vi "SET_8BITS_Command.vi"(9 "Valor en 8 bits":u8, 10 "Marca":T1) -> (1 "length":i32, 2 "Expected Response":string, 3 "Command":string, 4 "Bytes Expected":u32=2)   [LabVIEW 2019, in "Serial Device.lvclass"]
uses:
  Serial Device.lvclass
  Marca.ctl
  Comando.ctl
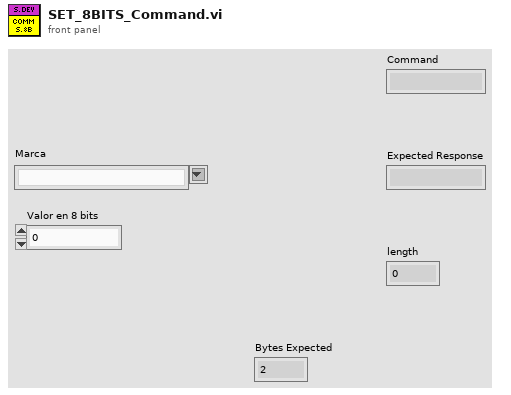
[diagram p1: front panel]
types:
  T1 = typedef "Marca.ctl" = string
  T2 = typedef "Comando.ctl" = string
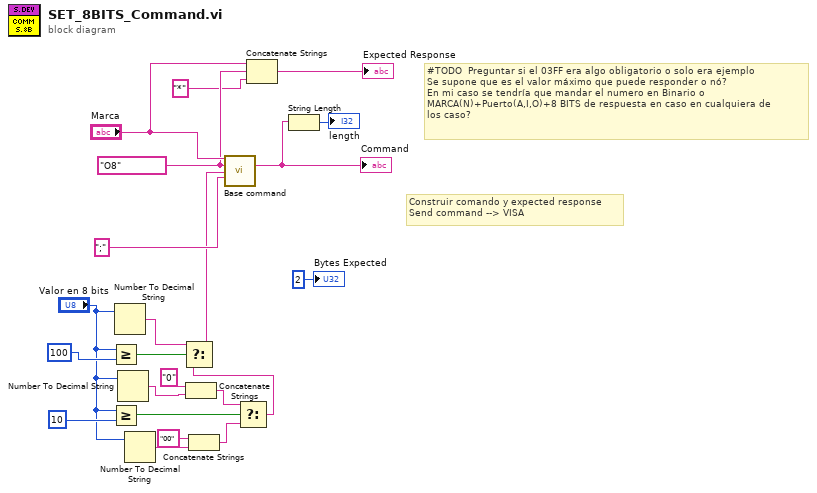
[diagram p0: block diagram]
diagram:
  w21 = T2 "O8" ("Comando")
  # "Construir comando y expected response\nSend command --> VISA"
  # "#TODO  Preguntar si el 03FF era algo obligatorio o solo era ejemplo\nSe supone que es el valor máximo que puede responder o nó?\nEn mi caso se tendría que mandar el numero en Binario o \nMARCA(N)+Puerto(A,I,O)+8 BITS de respuesta en caso en cualquiera de \nlos caso?"
  n1 = Greater Or Equal?(x="Valor en 8 bits", y=u8 100) -> (x >= y?=w12:bool)
  n2 = Greater Or Equal?(x="Valor en 8 bits", y=u8 10) -> (x >= y?=w7:bool)
  n3 = Number To Decimal String(number="Valor en 8 bits") -> (decimal integer string=w13:string)  [unwired: 1 in]
  n4 = Number To Decimal String(number="Valor en 8 bits") -> (decimal integer string=w9:string)  [unwired: 1 in]
  n5 = Number To Decimal String(number="Valor en 8 bits") -> (decimal integer string=w3:string)  [unwired: 1 in]
  n6 = Concatenate Strings("0" ("string"), w9) -> (w8:string)
  n7 = Concatenate Strings("00" ("string"), w3) -> (w5:string)
  n8 = Select(t=w8, s=w7, f=w5) -> (s? t:f=w2:string)
  n9 = Select(t=w13, s=w12, f=w2) -> (s? t:f=w1:string)
  n10 = call "Base command.vi"("Marca"="Marca", "Comando"=w21, "Parametro 1"=w1, "Parametro 2"=";") -> ("Command"=w19:string)  [unwired: 10 in, 1 out]
  "Command" <- w19
  n11 = Concatenate Strings("Marca", w21, "*") -> (→"Expected Response":string)
  n12 = String Length(string=w19) -> (length=→"length":i32)
  "Bytes Expected" <- u32 2 ("byte count")
